vi "Actor.vi"(10 "Error Q":refnum<queue>, 11 "Self Actor in":refnum<class "Self Actor.lvclass">) -> ()   [LabVIEW 2021, in "AAM.lvlib" / "Self Actor.lvclass"]
uses:
  Self Actor.lvclass
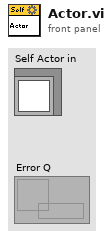
[diagram p1: front panel]
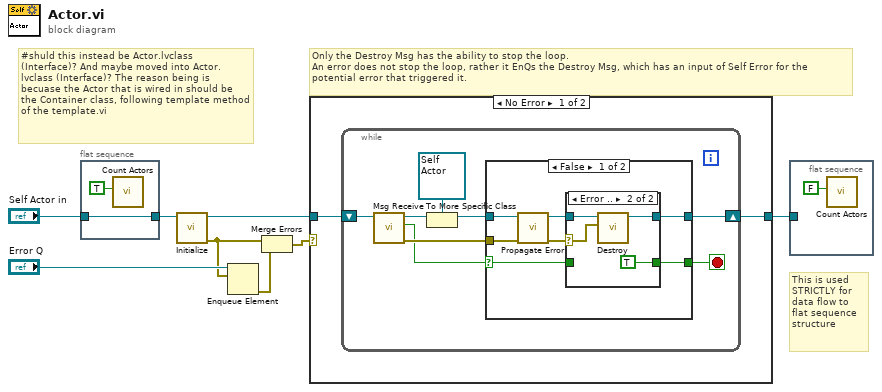
[diagram p0: block diagram]
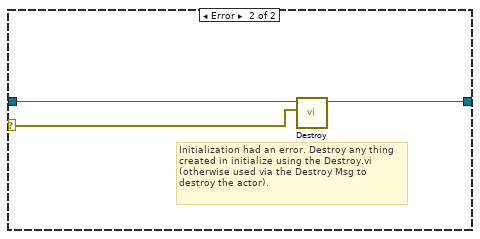
[diagram p4: hidden frame]
diagram:
  # "This is used STRICTLY for data flow to flat sequence structure"
  # "#shuld this instead be Actor.lvclass (Interface)? And maybe moved into Actor.lvclass (Interface)? The reason being is becuase the Actor that is wired in should be the Container class, following template method of the template.vi"
  # "Only the Destroy Msg has the ability to stop the loop.\nAn error does not stop the loop, rather it EnQs the Destroy Msg, which has an input of Self Error for the potential error that triggered it."
  n1 = flat-sequence {
    tunnel: [w9] -> w4
    tunnel: "Self Actor in" -> [w9]
    frame #0 {
      n2 = call "Count Actors.vi"("Increment?"=TRUE) -> ()  [unwired: 11 in]
    }
  }
  n3 = call-dynamic "Initialize.vi"("Self Actor in"=w4) -> ("error out"=w5:errorcluster, "Self Actor out"=w7:refnum<class "Self Actor.lvclass">)  [unwired: 9 in]
  n4 = Enqueue Element(queue="Error Q", element=w5) -> (error out=w1:errorcluster)  [unwired: 2 in, 2 out]
  n5 = Merge Errors(w5, w1) -> (w2:errorcluster)
  n6 = case shown="No Error" w2 {
    selector: w2 -> [_ w37]
    tunnel: w7 -> [w12 w38]
    tunnel: [w11 w36] -> w3
    frame No Error {
      n7 = while {
        shift-right: [w20] -> w11
        shift-left: w12 -> [w19]
        stop <- w13 stop-if-true
        n8 = call-dynamic "Msg Receive.vi"("Self Actor in"=w19) -> ("error out"=w15:errorcluster, "Destroy Self?"=w14:bool, "Actor out"=w18:refnum<class "Actor.lvclass">)  [unwired: 8 in]
        n9 = To More Specific Class(target class=refnum<class "Self Actor.lvclass"> refnum ("Artifex Actor Model.lvlib:Self Actor.lvclass"), reference=w18) -> (specific class reference=w17:refnum<class "Self Actor.lvclass">)  [unwired: 1 in, 1 out]
        n10 = case shown="False" w14 {
          selector: w14 -> [w21 w34]
          tunnel: w15 -> [w26 _]
          tunnel: [w24 w35] -> w20
          tunnel: w17 -> [w27 w35]
          tunnel: [w22 w34] -> w13
          frame False {
            n11 = call-dynamic "Propagate Error.vi"("error in (no error)"=w26, "Self Actor in"=w27) -> ("error out"=w25:errorcluster, "Self Actor out"=w23:refnum<class "Self Actor.lvclass">)  [unwired: 8 in]
            n12 = case shown="Error .." w25 {
              selector: w25 -> [_ w31]
              tunnel: [w29 w32] -> w24
              tunnel: w23 -> [w29 w33]
              tunnel: [w28 TRUE] -> w22
              tunnel: w21 -> [w28 _]
              frame No Error {
              }
              frame Error {
                n13 = call-dynamic "Destroy.vi"("Error"=w31, "Self Actor in"=w33) -> ("Self Actor out"=w32:refnum<class "Self Actor.lvclass">)  [unwired: 8 in, 1 out]
              }
            }
          }
          frame True {
          }
        }
      }
    }
    frame Error {
      # "Initialization had an error. Destroy any thing created in initialize using the Destroy.vi (otherwise used via the Destroy Msg to destroy the actor)."
      n14 = call-dynamic "Destroy.vi"("Error"=w37, "Self Actor in"=w38) -> ("Self Actor out"=w36:refnum<class "Self Actor.lvclass">)  [unwired: 8 in, 1 out]
    }
  }
  n15 = flat-sequence {
    tunnel: w3 -> [_]
    frame #0 {
      n16 = call "Count Actors.vi"("Increment?"=FALSE) -> ()  [unwired: 11 in]
    }
  }
